vi "Open Form Button.vi"(8 "error in (no error)":errorcluster, 9 "Class Path":path, 10 "Ctl Refnum":refnum<vi>, 11 "Open Form in":refnum<class "Open Form.lvclass">) -> (0 "error out":errorcluster, 3 "Open Form out":refnum<class "Open Form.lvclass">)   [LabVIEW 2020, in "Open Form Button.lvlib" / "Open Form.lvclass"]
uses:
  Open Form.lvclass
  C:/Users/User/Desktop/Raman Program/Database OOP/source/Button/Button Class/Button.lvclass
  Button/Button Class/Button.lvclass/Button.ctl
  Open Form.lvclass/Open Form.ctl
  Button/Button Class/Button.lvclass
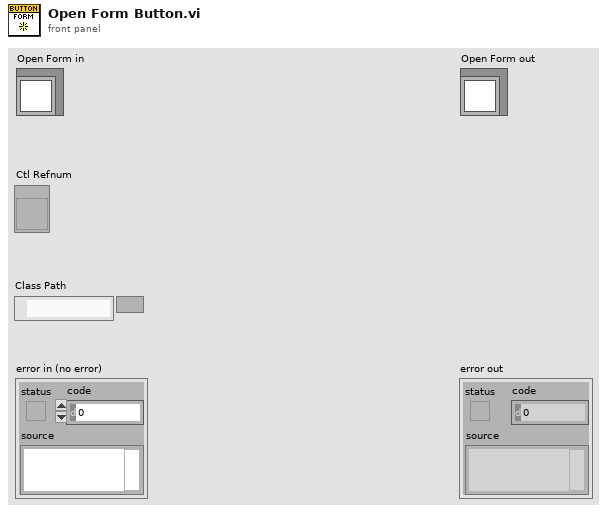
[diagram p1: front panel]
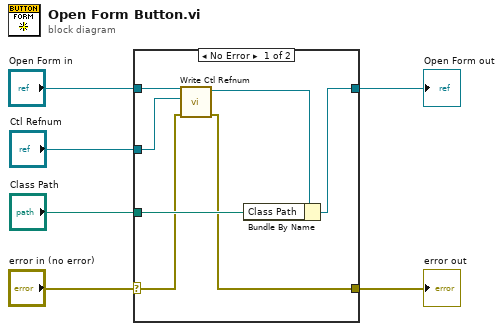
[diagram p0: block diagram]
diagram:
  n1 = case shown="No Error" "error in (no error)" {
    selector: "error in (no error)" -> [w8 w15]
    tunnel: [w7 w15] -> w5
    tunnel: [w10 w14] -> w3
    tunnel: "Open Form in" -> [w13 w14]
    tunnel: "Ctl Refnum" -> [w12 _]
    tunnel: "Class Path" -> [w9 _]
    frame No Error {
      n2 = call "Write Ctl Refnum.vi"("error in (no error)"=w8, "Ctl Refnum"=w12, "Button in"=w13) -> ("error out"=w7:errorcluster, "Button out"=w11:refnum<class "Open Form.lvclass">)  [unwired: 7 in]
      n3 = Bundle By Name(cluster=w11, "Class Path"=w9) -> (w10:refnum<class "Open Form.lvclass">)
    }
    frame Error {
    }
  }
  "error out" <- w5
  "Open Form out" <- w3
